vi "Add Dependencies.vi"(8 "error in (no error)":errorcluster, 10 "Dependencies":refnum<class "PackageAbstract.lvclass">[](array[class]), 11 "PackageAbstract in":refnum<class "PackageAbstract.lvclass">) -> (0 "error out":errorcluster, 3 "PackageAbstract out":refnum<class "PackageAbstract.lvclass">)   [LabVIEW 2020, in "GPack.lvlib" / "PackageAbstract.lvclass"]
uses:
  PackageAbstract.lvclass
  C:/dev/lv20CE/lv-gpack/GPack/Package/Package.lvclass
  Package Order.ctl
  Package/Package.lvclass
  PackageAbstract.lvclass/PackageAbstract.ctl
  <vilib>/Utility/miscctls.llb/LVMapReplaceAction.ctl
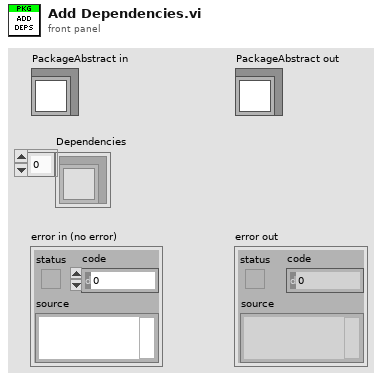
[diagram p1: front panel]
types:
  T1 = typedef "GPack.lvlib/PackageAbstract.lvclass/Package Order.ctl" = cluster{"Order":i32, "Pkg":refnum<class "Package.lvclass">}
  T2 = cluster{i32, "GPack.lvlib:Package.lvclass":refnum<class "Package.lvclass">}
  T3 = typedef "LVMapReplaceAction.ctl" = enum32{"Modify Entry only if found", "Add or Modify Entry", "Delete Entry"}
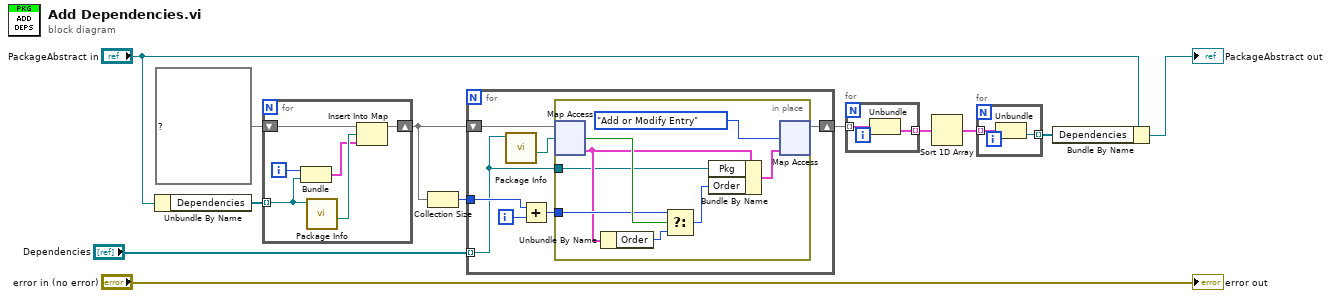
[diagram p0: block diagram]
diagram:
  n1 = Unbundle By Name("PackageAbstract in") -> ("Dependencies"=w11:refnum<class "Package.lvclass">[])
  n2 = for {
    tunnel: w11 -> [w16] mode=indexing
    shift-right: [w13] -> w3
    shift-left: map{path, T1} {} ("map") -> [w15]
    i -> [w17]
    n3 = Bundle(w17, "GPack.lvlib:Package.lvclass"=w16) -> (w14:T2)  [unwired: 1 in]
    n4 = call-dynamic "Package Info.vi"("Package in"=w16) -> ("Folder"=w18:path)  [unwired: 8 in, 2 out]
    n5 = Insert Into Map(map in=w15, key=w18, value=w14) -> (map out=w13:map{path, T1})  [unwired: 2 out]
  }
  n6 = Collection Size(1:w3) -> (0:w9:i32)
  n7 = for {
    tunnel: "Dependencies" -> [w20] mode=indexing
    shift-right: [w21] -> w8
    shift-left: w3 -> [w25]
    tunnel: w9 -> [w24]
    i -> [w23]
    n8 = call-dynamic "Package Info.vi"("Package in"=w20) -> ("Folder"=w19:path)  [unwired: 8 in, 2 out]
    n9 = Add(x=w24, y=w23) -> (x+y=w22:i32)
    n10 = in-place {
      in-place-border: w20 -> [w28]
      in-place-border: w22 -> [w32]
      n11 = in-place-map #1(w25, w19) -> (w31:T1, w33:bool)  [unwired: 1 in]
      n12 = Unbundle By Name(w31) -> ("Order"=w30:i32)
      n13 = Select(t=w32, s=w33, f=w30) -> (s? t:f=w29:i32)
      n14 = Bundle By Name(cluster=w31, "Pkg"=w28, "Order"=w29) -> (w27:T1)
      n15 = in-place-map #1(w27, LVMapReplaceAction."Add or Modify Entry" ("action")) -> (w21:map{path, T1})  [unwired: 2 out]
    }
  }
  n16 = for {
    tunnel: w8 -> [w35] mode=indexing
    tunnel: [w34] -> w7 mode=indexing
    n17 = Unbundle(w35) -> ("Package Order"=w34:T1)  [unwired: 1 out]
  }
  n18 = Sort 1D Array(array=w7) -> (sorted array=w6:T1[])
  n19 = for {
    tunnel: w6 -> [w37] mode=indexing
    tunnel: [w36] -> w5 mode=indexing
    n20 = Unbundle(w37) -> ("Pkg"=w36:refnum<class "Package.lvclass">)  [unwired: 1 out]
  }
  n21 = Bundle By Name(cluster="PackageAbstract in", "Dependencies"=w5) -> (→"PackageAbstract out":refnum<class "PackageAbstract.lvclass">)
  "error out" <- "error in (no error)"
